vi "XNET Read (State CAN Comm).vi"(0 "session in":refnum<k21>, 11 "error in (no error)":errorcluster) -> (4 "session out":refnum<k21>, 6 "CAN comm":T1 {"fault code" format="%08x"; "last error" items=["None", "Stuff", "Form", "Ack", "Bit1", "Bit0", "CRC"]; "communication state" items=["Error Active", "Error Passive", "Bus Off", "Init"]}, 15 "error out":errorcluster)   [LabVIEW 2018]
doc: "Reads the state of CAN communication using an XNET session."
uses:
  XNET CAN Comm.ctl
  XNET CAN Comm State.ctl
  XNET CAN Last Err.ctl
  nixlvapi.dll
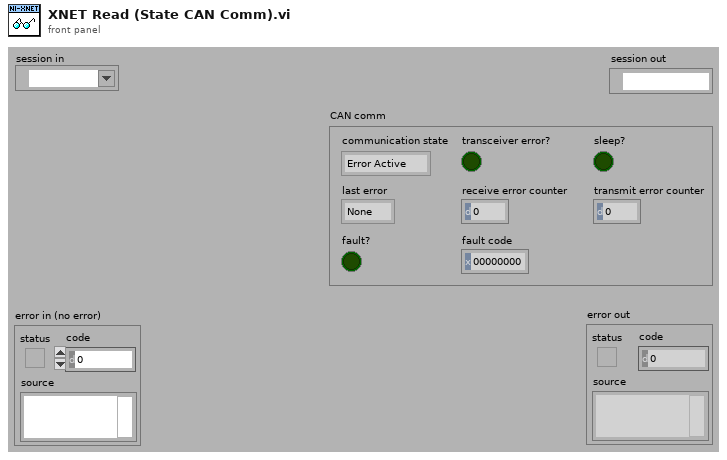
[diagram p1: front panel]
types:
  T1 = typedef "XNET CAN Comm.ctl" = cluster{"fault code":i32, "fault?":bool, "communication state":T2, "last error":T3, "receive error counter":u8, "transmit error counter":u8, "transceiver error?":bool, "sleep?":bool}
  T2 = typedef "XNET CAN Comm State.ctl" = u8
  T3 = typedef "XNET CAN Last Err.ctl" = u8
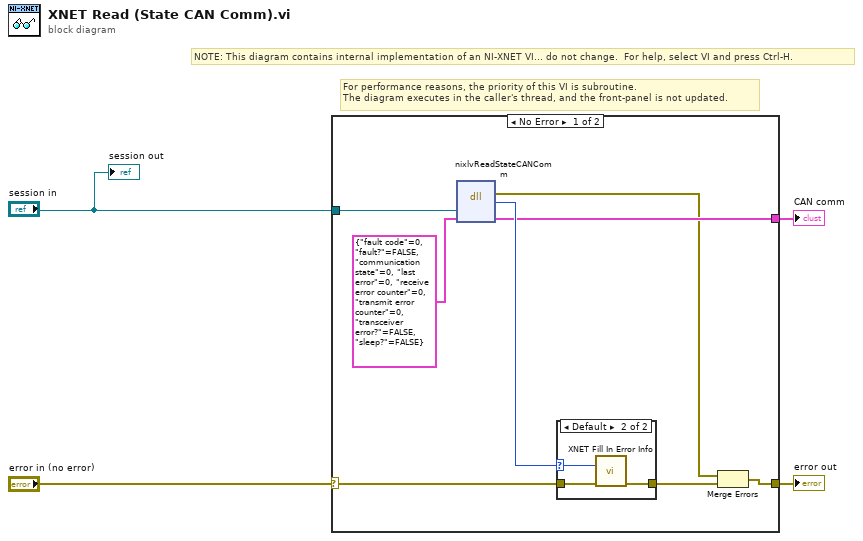
[diagram p0: block diagram]
diagram:
  # "For performance reasons, the priority of this VI is subroutine.\nThe diagram executes in the caller's thread, and the front-panel is not updated."
  # "NOTE: This diagram contains internal implementation of an NI-XNET VI... do not change.  For help, select VI and press Ctrl-H."
  n1 = case shown="No Error" "error in (no error)" {
    selector: "error in (no error)" -> [w11 w17]
    tunnel: "session in" -> [w12 _]
    tunnel: [w6 w17] -> w4
    tunnel: [w7 _] -> w1
    frame No Error {
      n2 = dll-call lib="nixlvapi.*" fn="nixlvReadStateCANComm"("sessionRef"=w12, "CANComm"=T1 {"fault code"=0, "fault?"=FALSE, "communication state"=0, "last error"=0, "receive error counter"=0, "transmit error counter"=0, "transceiver error?"=FALSE, "sleep?"=FALSE} ("CAN comm")) -> (error out=w5:errorcluster, "return type"=w9:i32, "CANComm"=w7:T1)  [unwired: 3 in, 2 out]
      n3 = case shown="Default" w9 {
        selector: w9 -> [_ w14]
        tunnel: w11 -> [w13 w15]
        tunnel: [w13 w16] -> w10
        frame 0 {
        }
        frame Default {
          n4 = call "XNET Fill In Error Info.vi"("status code"=w14, "error in"=w15) -> ("error out"=w16:errorcluster)  [unwired: 13 out]
        }
      }
      n5 = Merge Errors(w5, w10) -> (w6:errorcluster)
    }
    frame Error {
    }
  }
  "error out" <- w4
  "CAN comm" <- w1
  "session out" <- "session in"
